vi "Set_Gain_OE-200.vi"(3 "error in":errorcluster, 4 "Status":i32, 5 "Gain  [V/W]":T1(ring), 6 "index":i32) -> (0 "error out":errorcluster, 1 "Status_out":i32, 2 "index_out":i32)   [LabVIEW 2010, in "FEMTO_LUCI-10.lvlib"]
uses:
  <userlib>/FEMTO/FEMTO_LUCI-10.lvlib
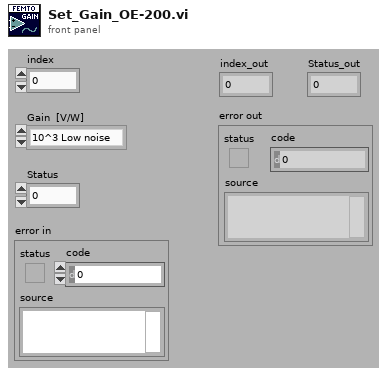
[diagram p1: front panel]
types:
  T1 = enum16{"10^3 Low noise", "10^4 Low noise", "10^5 Low noise", "10^6 Low noise", "10^7 Low noise", "10^8 Low noise", "10^9 Low noise", "10^5 High speed", "10^6 High speed", "10^7 High speed", "10^8 High speed", "10^9 High speed", "10^10 High speed", "10^11 High speed"}
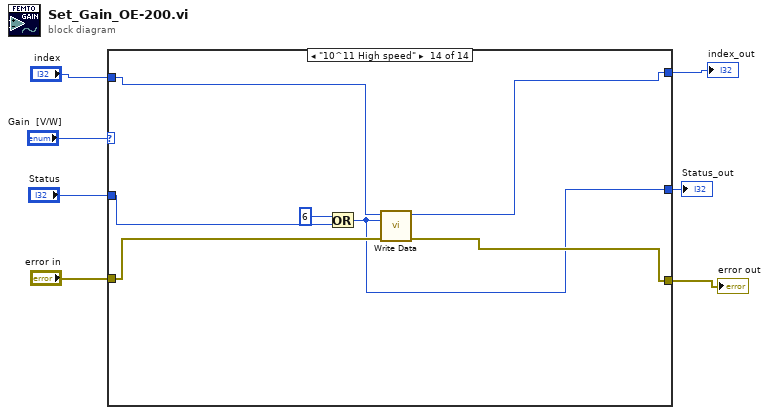
[diagram p0: block diagram]
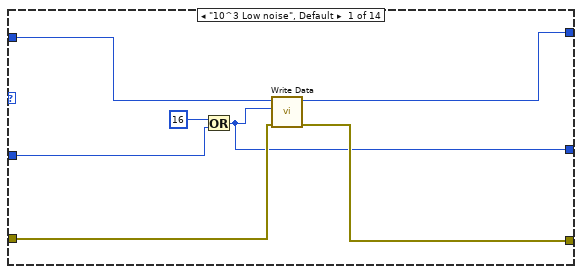
[diagram p2: hidden frame]
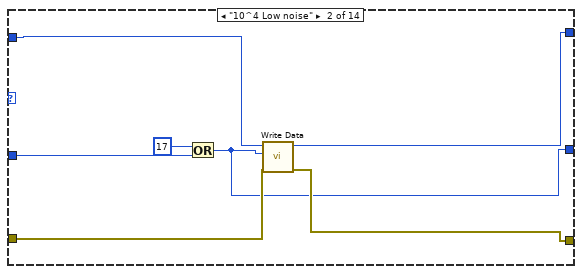
[diagram p3: hidden frame]
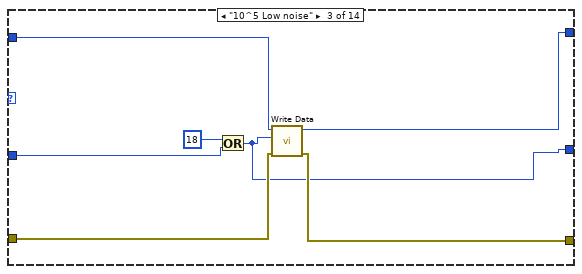
[diagram p4: hidden frame]
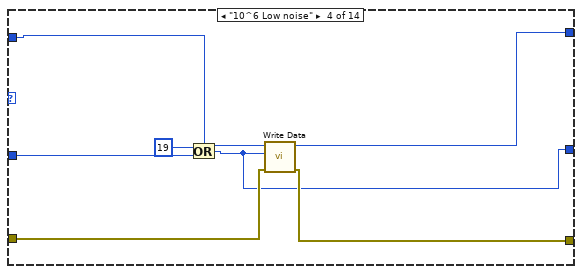
[diagram p5: hidden frame]
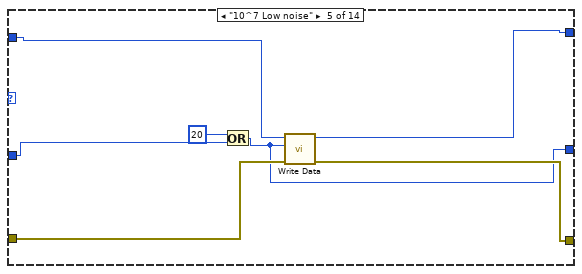
[diagram p6: hidden frame]
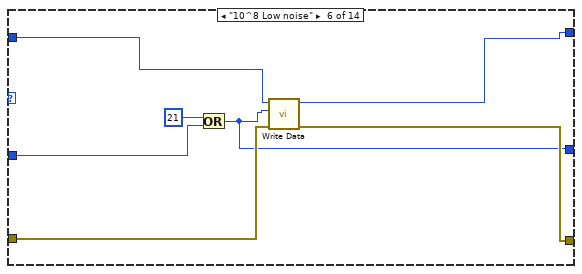
[diagram p7: hidden frame]
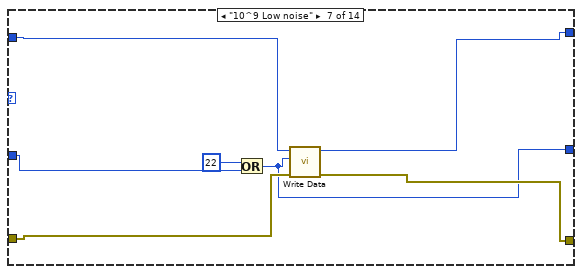
[diagram p8: hidden frame]
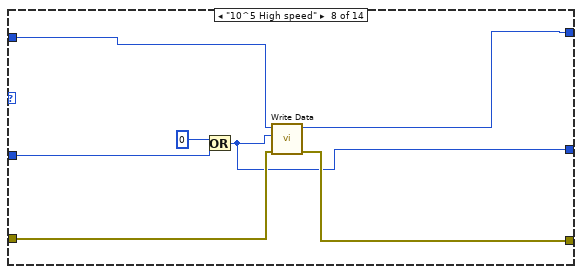
[diagram p9: hidden frame]
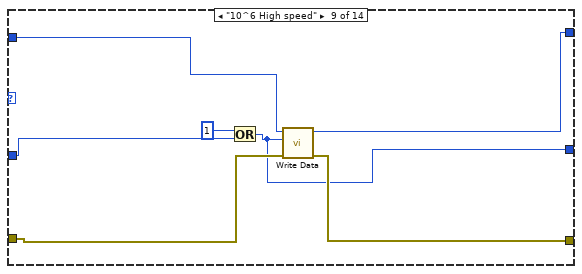
[diagram p10: hidden frame]
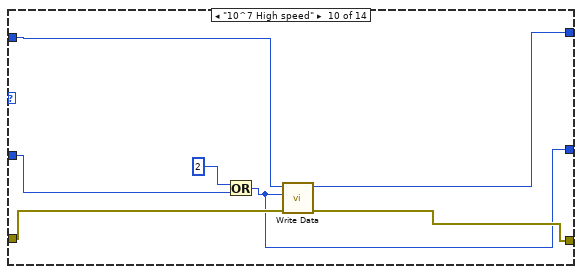
[diagram p11: hidden frame]
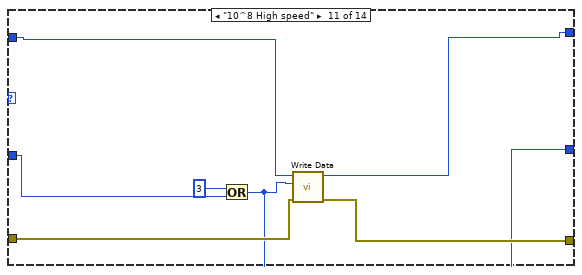
[diagram p12: hidden frame]
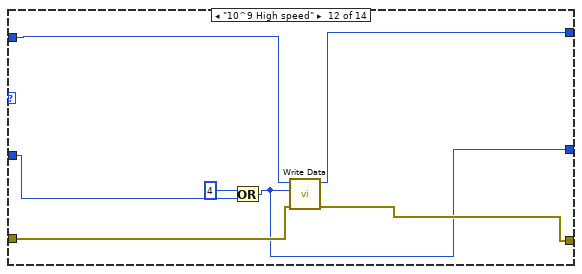
[diagram p13: hidden frame]
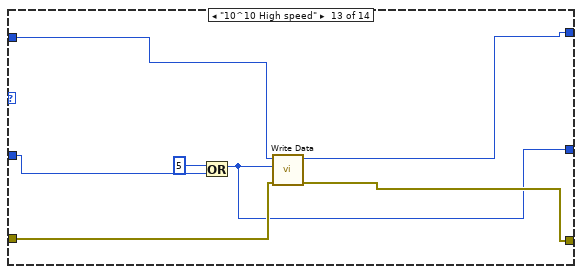
[diagram p14: hidden frame]
diagram:
  n1 = case shown="\"10^11 High speed\"" "Gain  [V/W]" {
    tunnel: "index" -> [w14 w18 w27 w33 w41 w49 w55 w62 w66 w73 w80 w86 w98 w104]
    tunnel: [w13 w17 w26 w32 w40 w48 w54 w61 w65 w74 w79 w87 w97 w103] -> w4
    tunnel: "error in" -> [w12 w20 w24 w30 w38 w45 w52 w59 w69 w76 w84 w89 w94 w101]
    tunnel: [w11 w19 w25 w31 w39 w44 w53 w58 w68 w75 w83 w88 w93 w102] -> w6
    tunnel: "Status" -> [w9 w16 w23 w34 w37 w46 w51 w60 w67 w72 w81 w90 w95 w100]
    tunnel: [w8 w15 w22 w29 w36 w43 w50 w57 w64 w71 w78 w85 w92 w99] -> w1
    frame "10^3 Low noise", Default {
      n2 = Or(x=16 ("data_low"), y=w9) -> (x .or. y?=w8:i32)
      n3 = call <userlib>:"Write Data.vi"("error in (no error)"=w12, "data_low"=w8, "index"=w14) -> ("error out"=w11:errorcluster, "index_out"=w13:i32)  [unwired: 1 in, 6 out]
    }
    frame "10^4 Low noise" {
      n4 = Or(x=17 ("data_low"), y=w16) -> (x .or. y?=w15:i32)
      n5 = call <userlib>:"Write Data.vi"("error in (no error)"=w20, "data_low"=w15, "index"=w18) -> ("error out"=w19:errorcluster, "index_out"=w17:i32)  [unwired: 1 in, 6 out]
    }
    frame "10^5 Low noise" {
      n6 = Or(x=18 ("data_low"), y=w23) -> (x .or. y?=w22:i32)
      n7 = call <userlib>:"Write Data.vi"("error in (no error)"=w24, "data_low"=w22, "index"=w27) -> ("error out"=w25:errorcluster, "index_out"=w26:i32)  [unwired: 1 in, 6 out]
    }
    frame "10^6 Low noise" {
      n8 = Or(x=19 ("data_low"), y=w34) -> (x .or. y?=w29:i32)
      n9 = call <userlib>:"Write Data.vi"("error in (no error)"=w30, "data_low"=w29, "index"=w33) -> ("error out"=w31:errorcluster, "index_out"=w32:i32)  [unwired: 1 in, 6 out]
    }
    frame "10^7 Low noise" {
      n10 = Or(x=20 ("data_low"), y=w37) -> (x .or. y?=w36:i32)
      n11 = call <userlib>:"Write Data.vi"("error in (no error)"=w38, "data_low"=w36, "index"=w41) -> ("error out"=w39:errorcluster, "index_out"=w40:i32)  [unwired: 1 in, 6 out]
    }
    frame "10^8 Low noise" {
      n12 = Or(x=21 ("data_low"), y=w46) -> (x .or. y?=w43:i32)
      n13 = call <userlib>:"Write Data.vi"("error in (no error)"=w45, "data_low"=w43, "index"=w49) -> ("error out"=w44:errorcluster, "index_out"=w48:i32)  [unwired: 1 in, 6 out]
    }
    frame "10^9 Low noise" {
      n14 = Or(x=22 ("data_low"), y=w51) -> (x .or. y?=w50:i32)
      n15 = call <userlib>:"Write Data.vi"("error in (no error)"=w52, "data_low"=w50, "index"=w55) -> ("error out"=w53:errorcluster, "index_out"=w54:i32)  [unwired: 1 in, 6 out]
    }
    frame "10^5 High speed" {
      n16 = Or(x=0 ("data_low"), y=w60) -> (x .or. y?=w57:i32)
      n17 = call <userlib>:"Write Data.vi"("error in (no error)"=w59, "data_low"=w57, "index"=w62) -> ("error out"=w58:errorcluster, "index_out"=w61:i32)  [unwired: 1 in, 6 out]
    }
    frame "10^6 High speed" {
      n18 = Or(x=1 ("data_low"), y=w67) -> (x .or. y?=w64:i32)
      n19 = call <userlib>:"Write Data.vi"("error in (no error)"=w69, "data_low"=w64, "index"=w66) -> ("error out"=w68:errorcluster, "index_out"=w65:i32)  [unwired: 1 in, 6 out]
    }
    frame "10^7 High speed" {
      n20 = Or(x=2 ("data_low"), y=w72) -> (x .or. y?=w71:i32)
      n21 = call <userlib>:"Write Data.vi"("error in (no error)"=w76, "data_low"=w71, "index"=w73) -> ("error out"=w75:errorcluster, "index_out"=w74:i32)  [unwired: 1 in, 6 out]
    }
    frame "10^8 High speed" {
      n22 = Or(x=3 ("data_low"), y=w81) -> (x .or. y?=w78:i32)
      n23 = call <userlib>:"Write Data.vi"("error in (no error)"=w84, "data_low"=w78, "index"=w80) -> ("error out"=w83:errorcluster, "index_out"=w79:i32)  [unwired: 1 in, 6 out]
    }
    frame "10^9 High speed" {
      n24 = Or(x=4 ("data_low"), y=w90) -> (x .or. y?=w85:i32)
      n25 = call <userlib>:"Write Data.vi"("error in (no error)"=w89, "data_low"=w85, "index"=w86) -> ("error out"=w88:errorcluster, "index_out"=w87:i32)  [unwired: 1 in, 6 out]
    }
    frame "10^10 High speed" {
      n26 = Or(x=5 ("data_low"), y=w95) -> (x .or. y?=w92:i32)
      n27 = call <userlib>:"Write Data.vi"("error in (no error)"=w94, "data_low"=w92, "index"=w98) -> ("error out"=w93:errorcluster, "index_out"=w97:i32)  [unwired: 1 in, 6 out]
    }
    frame "10^11 High speed" {
      n28 = Or(x=6 ("data_low"), y=w100) -> (x .or. y?=w99:i32)
      n29 = call <userlib>:"Write Data.vi"("error in (no error)"=w101, "data_low"=w99, "index"=w104) -> ("error out"=w102:errorcluster, "index_out"=w103:i32)  [unwired: 1 in, 6 out]
    }
  }
  "index_out" <- w4
  "error out" <- w6
  "Status_out" <- w1
